vi "AI Inputs -- constant.vi"() -> (2 "AI Inputs":string[](array[string])=["DI0", "DI1", "DI2", "DI3", "DI4", "DI5", "DI6", "DI7", "DI8", "DI9", "DI10", "DI11", "DI12", "DI13", "DI14", "DI15"])   [LabVIEW 2019, in "TDMS.lvlib"]
uses:
  TDMS.lvlib
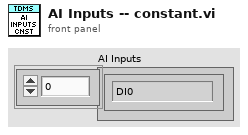
[diagram p1: front panel]
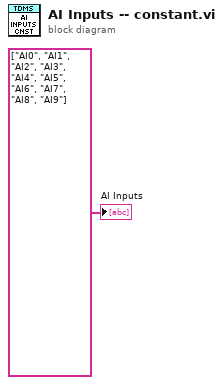
[diagram p0: block diagram]
diagram:
  "AI Inputs" <- string[] ["AI0", "AI1", "AI2", "AI3", "AI4", "AI5", "AI6", "AI7", "AI8", "AI9"]
